vi "SubMain1_WriteEEPROM_vna_wmg.vi"(6 "Date":u8[](array[numeric])=[49, 53, 48, 56, 50, 52] format="%.0x", 7 "VendorSN":u8[](array[numeric])=[49, 53, 50, 51, 54, 48, 48, 48, 53] format="%.0x", 8 "PN":string="H3C QSFP+", 9 "命令类型选择":string="H3C QSFP+", 10 "local":bool, 11 "VISA resource name":refnum<visa-resource-name>="COM1") -> (0 "cmd_input":string[][](array[string]), 1 "readout":string[][](array[string]), 2 "readout":u8[][](array[numeric]) format="%.0x", 3 "info_write":string[][](array[string]), 4 "type_array":string[](array[string]), 5 "exist?":bool)   [LabVIEW 2011]
uses:
  <vilib>/Utility/file.llb/Read From Spreadsheet File (string).vi
panel:
  out "output":string[][](array[string])
  out "电子表格字符串":string
  out "ext_array":string[][](array[string])
  out "ref_random":refnum<vi>
  in  "random":string[](array[string])
  out "ref_channel":refnum<vi>
  in  "channel":i8
  out "EEPROM_OK?":bool[](array[boolean])
  out "message":string
  # "EEPROM Information Output"
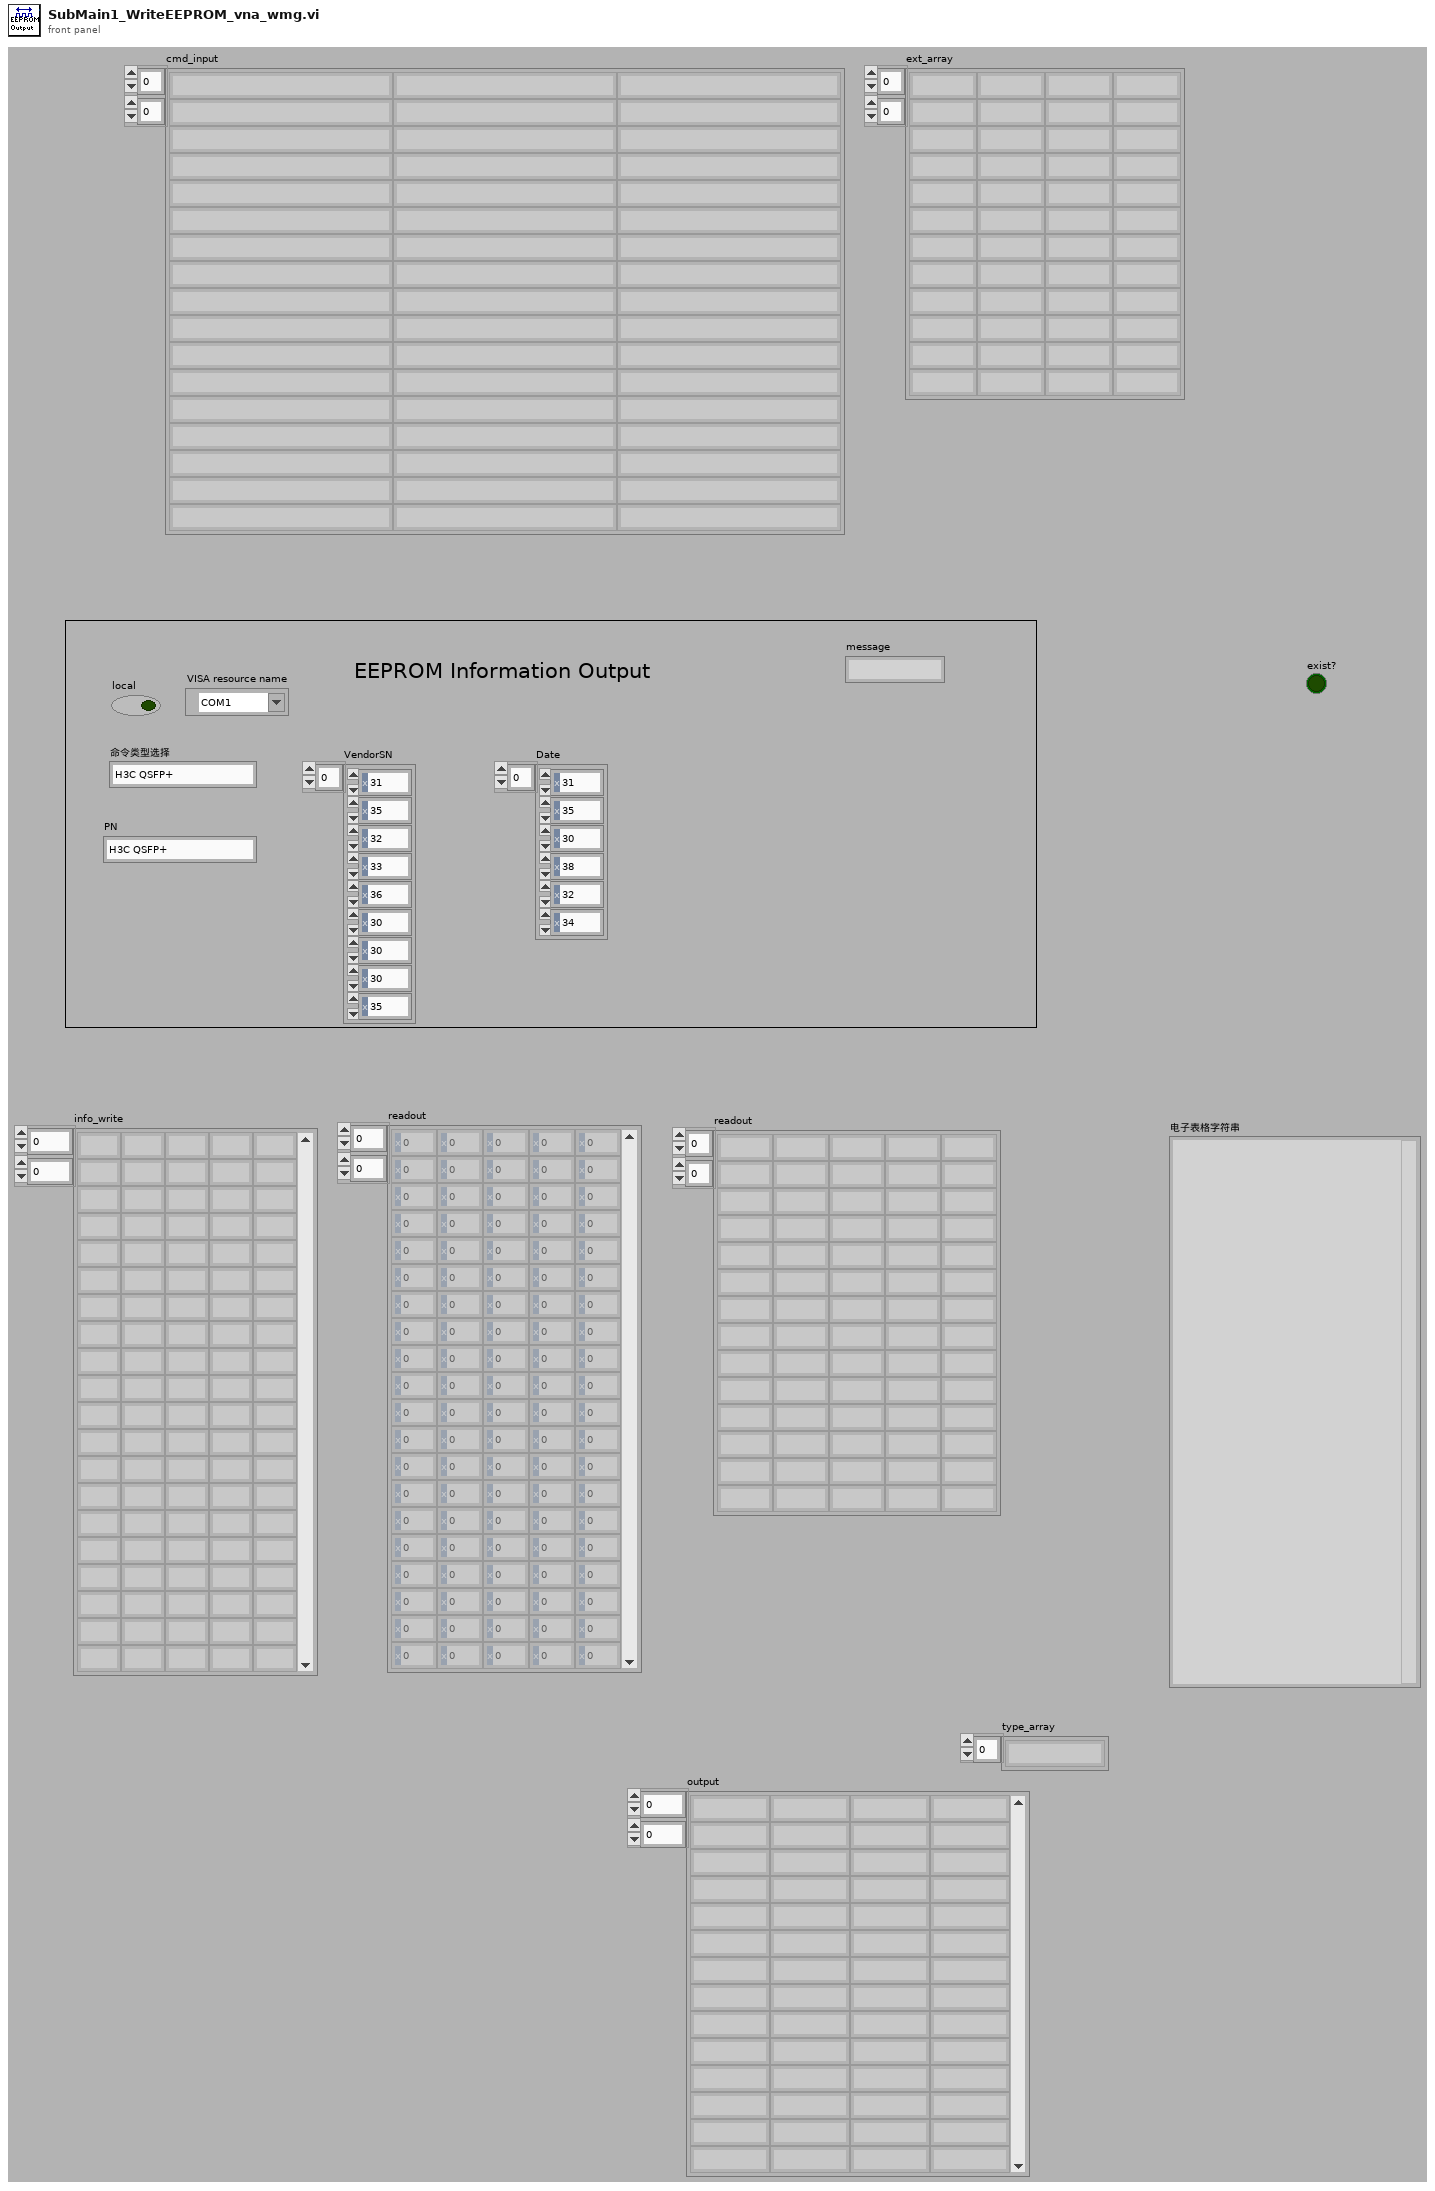
[diagram p1: front panel]
types:
  T1 = enum16{"查询表名", "查询列名", "查询记录", "查询总记录", "查询数据", "转换数据"}
  T2 = enum16{"big-endian, network order", "native, host order", "little-endian"}
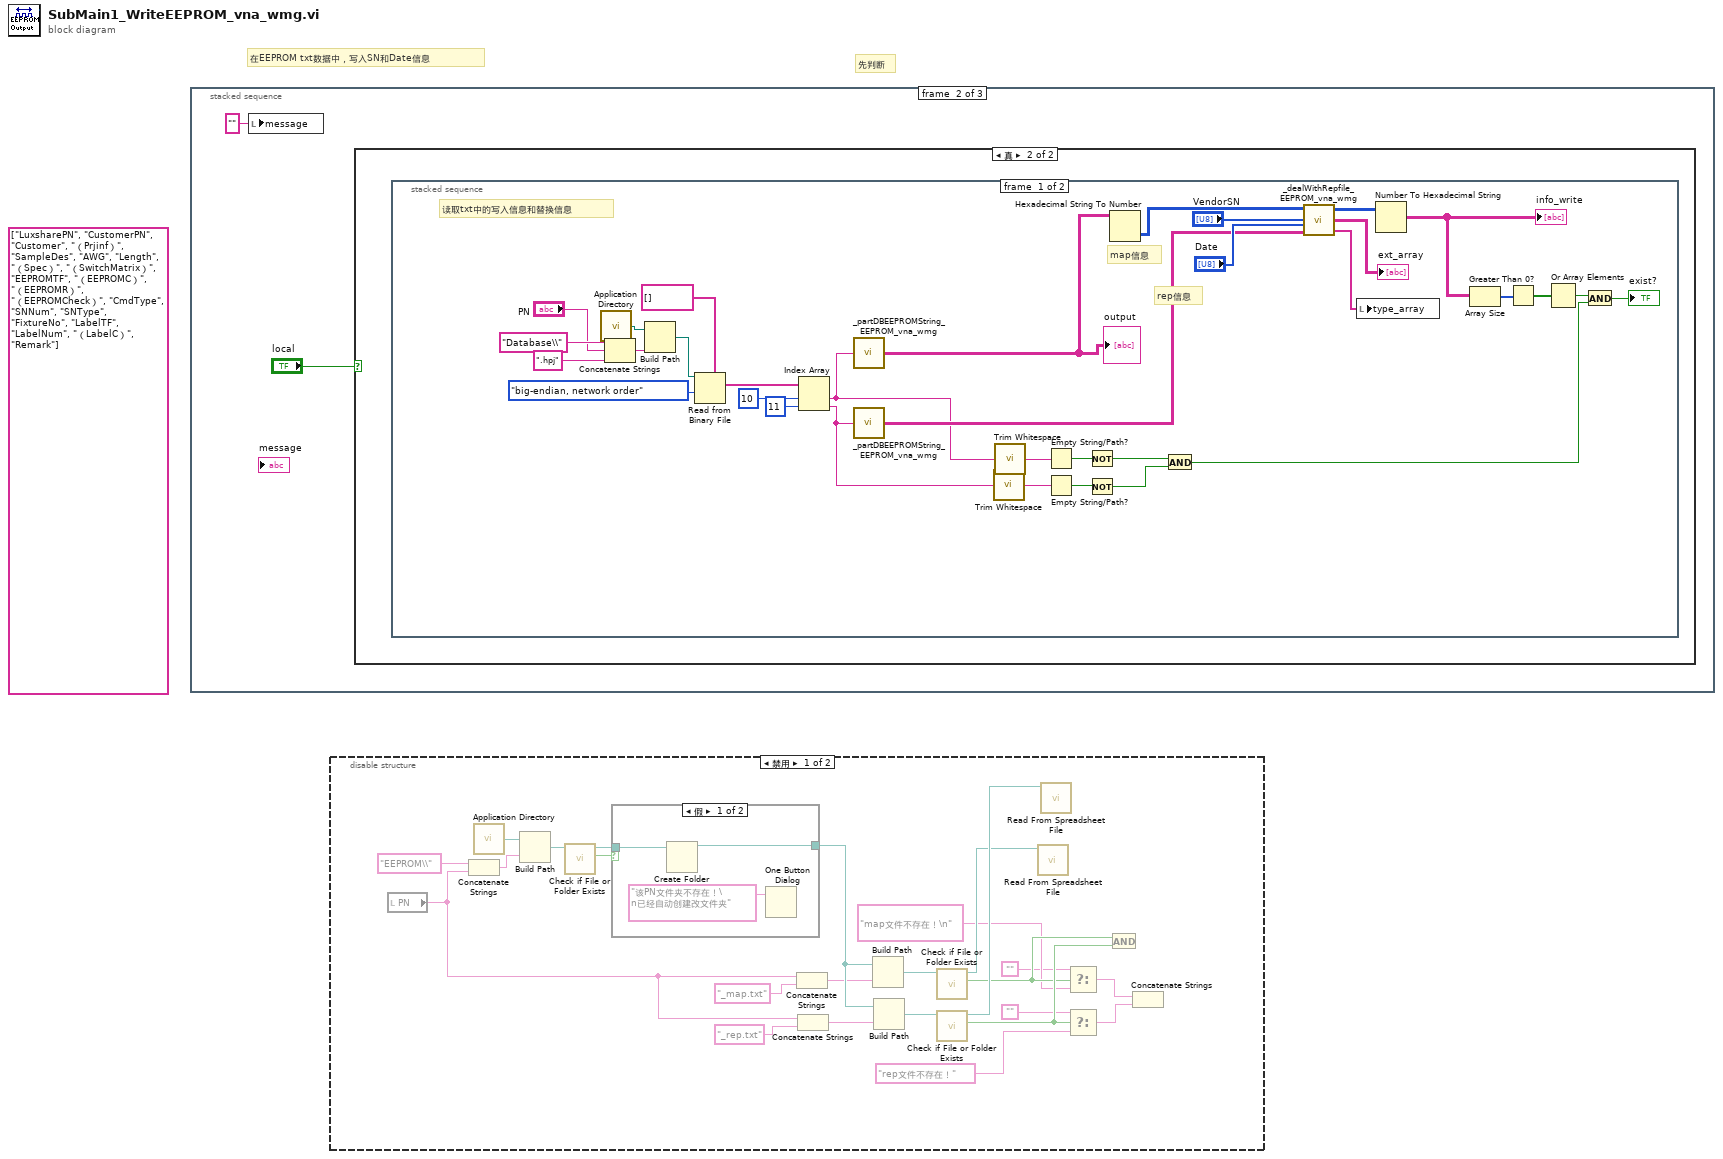
[diagram p0: block diagram]
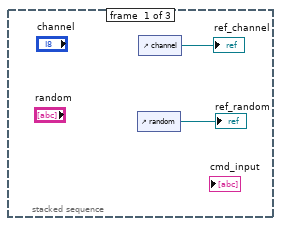
[diagram p4: hidden frame]
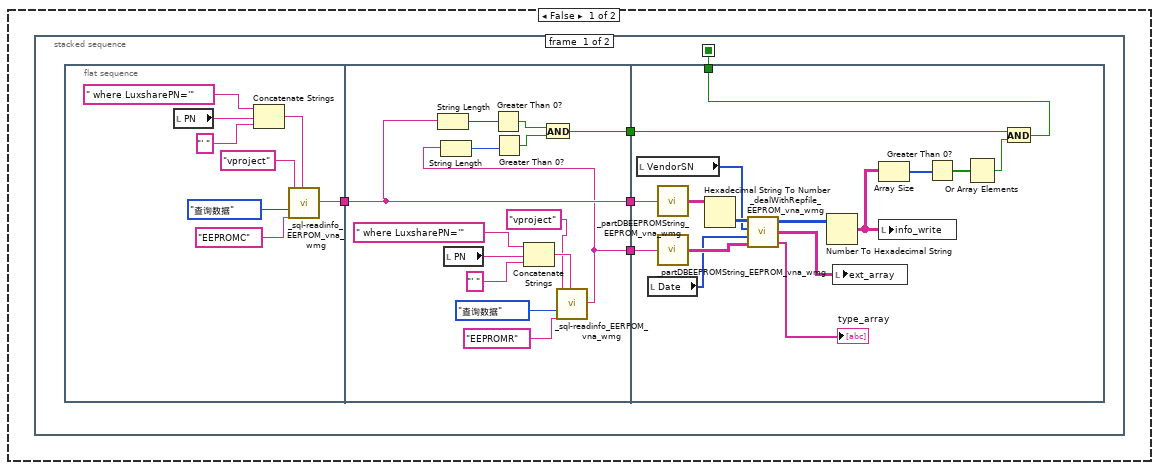
[diagram p5: hidden frame]
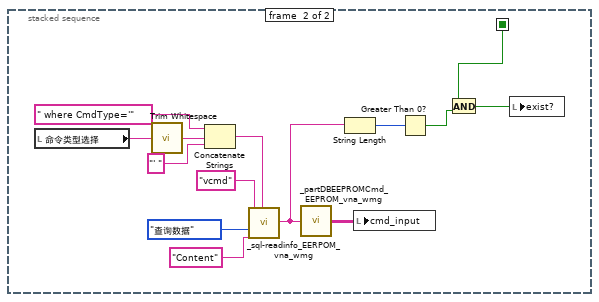
[diagram p6: hidden frame]
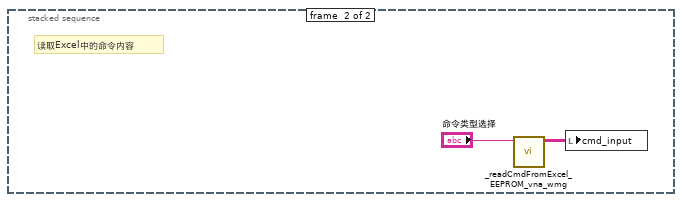
[diagram p7: hidden frame]
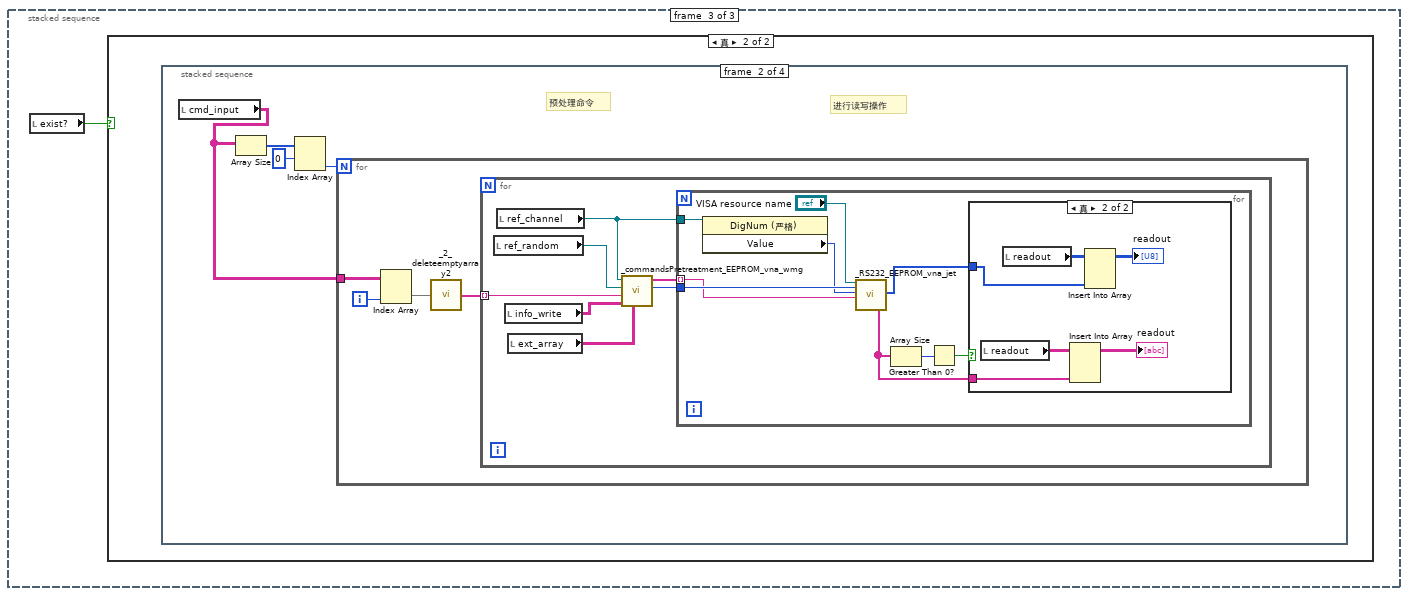
[diagram p8: hidden frame]
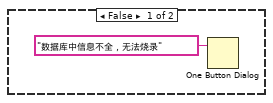
[diagram p9: hidden frame]
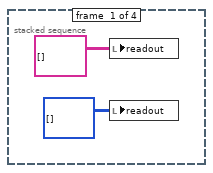
[diagram p10: hidden frame]
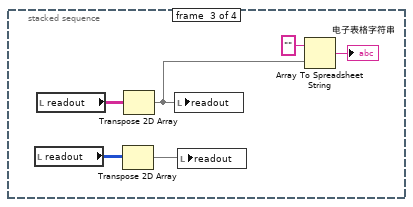
[diagram p12: hidden frame]
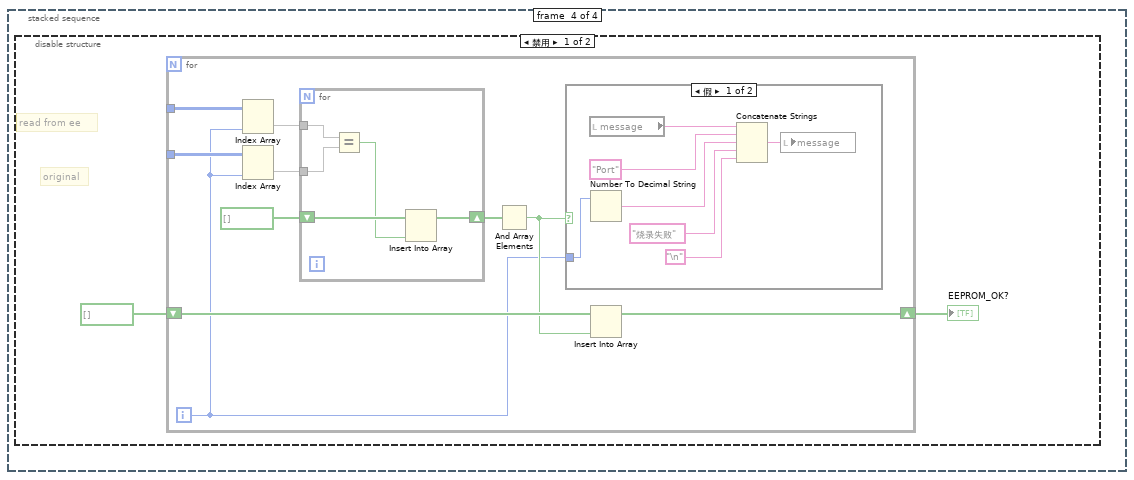
[diagram p13: hidden frame]
diagram:
  (unwired) string[] ["LuxsharePN", "CustomerPN", "Customer", "（Prjinf）", "SampleDes", "AWG", "Length", "（Spec）", "（SwitchMatrix）", "EEPROMTF", "（EEPROMC）", "（EEPROMR）", "（EEPROMCheck）", "CmdType", "SNNum", "SNType", "FixtureNo", "LabelTF", "LabelNum", "（LabelC）", "Remark"] ("列名")
  # "在EEPROM txt数据中，写入SN和Date信息"
  # "先判断"
  n1 = stacked-sequence {
    frame #0 {
      n2 = control-ref of="random"() -> (→"ref_random":refnum<vi>)
      n3 = control-ref of="channel"() -> (→"ref_channel":refnum<vi>)
    }
    frame #1 {
      n4 = local write "message"("" ("message")) -> ()
      n5 = case shown="真" "local" {
        frame False {
          n6 = stacked-sequence {
            seq-local: [w5 _] -> [_ w49]
            frame #0 {
              n7 = flat-sequence {
                tunnel: [w11] -> w9
                tunnel: w9 -> [w25]
                tunnel: [w25] -> w8
                tunnel: [w24] -> w7
                tunnel: [w19] -> w6
                tunnel: w8 -> [w47]
                tunnel: w7 -> [w46]
                tunnel: w6 -> [w37]
                tunnel: [w36] -> w5
                frame #0 {
                  n8 = local read "PN"() -> (w16:string)
                  n9 = Concatenate Strings(" where LuxsharePN='", w16, "' ") -> (w13:string)
                  n10 = call "_sql-readinfo_EERPOM_vna_wmg.vi"("操作模式"=T1."查询数据", "查询项目"="EEPROMC", "表名"="vproject", "限定条件"=w13) -> ("ResultString"=w11:string)  [unwired: 13 in, 10 out]
                }
                frame #1 {
                  n11 = String Length(string=w25) -> (length=w23:i32)
                  n12 = local read "PN"() -> (w27:string)
                  n13 = Greater Than 0?(x=w23) -> (x > 0?=w21:bool)
                  n14 = Concatenate Strings(" where LuxsharePN='", w27, "' ") -> (w30:string)
                  n15 = call "_sql-readinfo_EERPOM_vna_wmg.vi"("操作模式"=T1."查询数据", "查询项目"="EEPROMR", "表名"="vproject", "限定条件"=w30) -> ("ResultString"=w24:string)  [unwired: 13 in, 10 out]
                  n16 = String Length(string=w24) -> (length=w22:i32)
                  n17 = Greater Than 0?(x=w22) -> (x > 0?=w20:bool)
                  n18 = And(x=w21, y=w20) -> (x .and. y?=w19:bool)
                }
                frame #2 {
                  n19 = local read "VendorSN"() -> (w40:u8[])
                  n20 = local read "Date"() -> (w39:u8[])
                  n21 = call "_partDBEEPROMString_EEPROM_vna_wmg.vi"("input"=w47) -> ("output"=w44:string[][])
                  n22 = call "_partDBEEPROMString_EEPROM_vna_wmg.vi"("input"=w46) -> ("output"=w42:string[][])
                  n23 = Hexadecimal String To Number(string=w44) -> (number=w43:u32[][])  [unwired: 2 in, 1 out]
                  n24 = call "_dealWithRepfile_EEPROM_vna_wmg.vi"("eeprom_map"=w43, "VendorSN"=w40, "Date"=w39, "eeprom_rep"=w42) -> ("eeprom_map_out"=w45:u8[][], "ext_array"=w41:string[][], "type_array"=→"type_array":string[])  [unwired: 1 in]
                  n25 = Number To Hexadecimal String(2:w45) -> (0:w35:string[][])  [unwired: 1 in]
                  n26 = local write "ext_array"(w41) -> ()
                  n27 = Array Size(array=w35) -> (size(s)=w34:i32[])
                  n28 = local write "info_write"(w35) -> ()
                  n29 = Greater Than 0?(x=w34) -> (x > 0?=w33:bool[])
                  n30 = Or Array Elements(Boolean array=w33) -> (logical OR=w32:bool)
                  n31 = And(x=w37, y=w32) -> (x .and. y?=w36:bool)
                }
              }
            }
            frame #1 {
              n32 = local read "命令类型选择"() -> (w54:string)
              n33 = call <vilib>:"Trim Whitespace.vi"("string"=w54) -> ("trimmed string"=w55:string)  [unwired: 1 in]
              n34 = Concatenate Strings(" where CmdType='", w55, "' ") -> (w60:string)
              n35 = call "_sql-readinfo_EERPOM_vna_wmg.vi"("操作模式"=T1."查询数据", "查询项目"="Content", "表名"="vcmd", "限定条件"=w60) -> ("ResultString"=w52:string)  [unwired: 13 in, 10 out]
              n36 = call "_partDBEEPROMCmd_EEPROM_vna_wmg.vi"("input"=w52) -> ("output"=w53:string[][])
              n37 = String Length(string=w52) -> (length=w51:i32)
              n38 = local write "cmd_input"(w53) -> ()
              n39 = Greater Than 0?(x=w51) -> (x > 0?=w50:bool)
              n40 = And(x=w49, y=w50) -> (x .and. y?=w48:bool)
              n41 = local write "exist?"(w48) -> ()
            }
          }
        }
        frame True {
          n42 = stacked-sequence {
            frame #0 {
              # "map信息"
              # "rep信息"
              # "读取txt中的写入信息和替换信息"
              n43 = call <vilib>:"Application Directory.vi"() -> ("Application Directory"=w76:path)
              n44 = Concatenate Strings("Database\\" ("字符串"), "PN", ".hpj" ("字符串")) -> (w77:string)
              n45 = Build Path(base path=w76, name or relative path=w77) -> (appended path=w82:path)
              n46 = Read from Binary File(5:string[] [], 9:T2."big-endian, network order" ("字节顺序(0:big-endian, network order)"), 11:w82) -> (2:w83:string[])  [unwired: 3 in, 3 out]
              n47 = Index Array(array=w83, index #1=10 ("索引"), index #2=11 ("索引")) -> (element #1=w69:string, element #2=w68:string)
              n48 = call "_partDBEEPROMString_EEPROM_vna_wmg.vi"("input"=w69) -> ("output"=w62:string[][])
              "output" <- w62
              n49 = call "_partDBEEPROMString_EEPROM_vna_wmg.vi"("input"=w68) -> ("output"=w72:string[][])
              n50 = call <vilib>:"Trim Whitespace.vi"("string"=w68) -> ("trimmed string"=w70:string)  [unwired: 1 in]
              n51 = call <vilib>:"Trim Whitespace.vi"("string"=w69) -> ("trimmed string"=w71:string)  [unwired: 1 in]
              n52 = Empty String/Path?(string/path=w71) -> (empty?=w67:bool)
              n53 = Empty String/Path?(string/path=w70) -> (empty?=w66:bool)
              n54 = Not(x=w67) -> (.not. x?=w65:bool)
              n55 = Not(x=w66) -> (.not. x?=w64:bool)
              n56 = Hexadecimal String To Number(string=w62) -> (number=w84:u32[][])  [unwired: 2 in, 1 out]
              n57 = And(x=w65, y=w64) -> (x .and. y?=w63:bool)
              n58 = call "_dealWithRepfile_EEPROM_vna_wmg.vi"("eeprom_map"=w84, "VendorSN"="VendorSN", "Date"="Date", "eeprom_rep"=w72) -> ("eeprom_map_out"=w94:u8[][], "ext_array"=→"ext_array":string[][], "type_array"=w90:string[])  [unwired: 1 in]
              n59 = local write "type_array"(w90) -> ()
              n60 = Number To Hexadecimal String(2:w94) -> (0:w85:string[][])  [unwired: 1 in]
              "info_write" <- w85
              n61 = Array Size(array=w85) -> (size(s)=w88:i32[])
              n62 = Greater Than 0?(x=w88) -> (x > 0?=w87:bool[])
              n63 = Or Array Elements(Boolean array=w87) -> (logical OR=w86:bool)
              n64 = And(x=w86, y=w63) -> (x .and. y?=→"exist?":bool)
            }
            frame #1 {
              # "读取Excel中的命令内容"
              n65 = call "_readCmdFromExcel_EEPROM_vna_wmg.vi"("命令类型选择"="命令类型选择") -> ("cmd"=w95:string[][])  [unwired: 10 in]
              n66 = local write "cmd_input"(w95) -> ()
            }
          }
        }
      }
    }
    frame #2 {
      n67 = local read "exist?"() -> (w97:bool)
      n68 = case shown="真" w97 {
        frame False {
          n69 = One Button Dialog(message="数据库中信息不全，无法烧录" ("消息")) -> ()  [unwired: 1 in, 1 out]
        }
        frame True {
          n70 = stacked-sequence {
            frame #0 {
              n71 = local write "readout"(string[][] []) -> ()
              n72 = local write "readout"(u8[][] [] ("readout")) -> ()
            }
            frame #1 {
              # "进行读写操作"
              # "预处理命令"
              n73 = local read "cmd_input"() -> (w101:string[][])
              n74 = Array Size(array=w101) -> (size(s)=w104:i32[])
              n75 = Index Array(array=w104, index #1=0 ("索引")) -> (element #2=w102:i32)  [unwired: 1 in, 1 out]
              n76 = for {
                N: w102 -> [_]
                tunnel: w101 -> [w108]
                i -> [w107]
                n77 = Index Array(array=w108, index (col)=w107) -> (element=w106:string[])  [unwired: 1 in]
                n78 = call "_2_deleteemptyarray2.vi"("input"=w106) -> ("in_cons"=w105:string[])
                n79 = for {
                  tunnel: w105 -> [w113] mode=indexing
                  n80 = local read "ref_random"() -> (w114:refnum<vi>)
                  n81 = local read "ref_channel"() -> (w111:refnum<vi>)
                  n82 = local read "info_write"() -> (w110:string[][])
                  n83 = local read "ext_array"() -> (w109:string[][])
                  n84 = call "_commandsPretreatment_EEPROM_vna_wmg.vi"("array1_input"=w109, "array0_input"=w110, "cmd_input"=w113, "ref_random"=w114, "ref_channel"=w111) -> ("Function"=w112:enum16{"Write to EEPROM", "Read From EEPROM"}, "cmd_output"=w115:string[])  [unwired: 5 in]
                  n85 = for {
                    tunnel: w115 -> [w123] mode=indexing
                    tunnel: w112 -> [w124]
                    tunnel: w111 -> [w122]
                    n86 = property class="DigNum (严格)"(reference=w122) -> ("Value"=w121:i8)  [unwired: 1 in, 2 out]
                    n87 = call "_RS232_EEPROM_vna_jet.vi"("VISA resource name"="VISA resource name", "Function"=w124, "Select channel"=w121, "input_cmd"=w123) -> (13:"readout"=w117:string[], 16:"readout"=w116:u8[])  [unwired: 9 in, 5 out]
                    n88 = Array Size(array=w117) -> (size(s)=w119:i32)
                    n89 = Greater Than 0?(x=w119) -> (x > 0?=w118:bool)
                    n90 = case shown="真" w118 {
                      tunnel: w117 -> [_ w129]
                      tunnel: w116 -> [_ w126]
                      frame False {
                      }
                      frame True {
                        n91 = local read "readout"() -> (w130:string[][])
                        n92 = local read "readout"() -> (w127:u8[][])
                        n93 = Insert Into Array(array=w130, new element=w129) -> (→"readout":string[][])  [unwired: 2 in]
                        n94 = Insert Into Array(array=w127, new element=w126) -> (→"readout":u8[][])  [unwired: 2 in]
                      }
                    }
                  }
                }
              }
            }
            frame #2 {
              n95 = local read "readout"() -> (w135:u8[][])
              n96 = local read "readout"() -> (w136:string[][])
              n97 = Transpose 2D Array(2D array=w135) -> (transposed array=w134:u8[][])
              n98 = Transpose 2D Array(2D array=w136) -> (transposed array=w133:string[][])
              n99 = local write "readout"(w133) -> ()
              n100 = local write "readout"(w134) -> ()
              n101 = Array To Spreadsheet String(array=w133, 3:"" ("格式字符串")) -> (spreadsheet string=→"电子表格字符串":string)  [unwired: 1 in]
            }
            frame #3 {
              n102 = disable-structure shown="禁用" {
                frame Disabled {
                  # "read from ee"
                  # "original"
                  n103 = for {
                    N: [_] -> w141
                    tunnel: [w151] -> w140
                    tunnel: [w150] -> w139
                    shift-right: [w144] -> w137
                    shift-left: bool[] [] -> [w145]
                    i -> [w142]
                    n104 = Index Array(array=w151, index (col)=w142) -> (element=w149)  [unwired: 1 in]
                    n105 = Index Array(array=w150, index (col)=w142) -> (element=w148)  [unwired: 1 in]
                    n106 = for {
                      tunnel: w149 -> [w163]
                      tunnel: w148 -> [w162]
                      shift-right: [w159] -> w146
                      shift-left: bool[] [] -> [w161]
                      n107 = Equal?(x=w163, y=w162) -> (x = y?=w160:bool)
                      n108 = Insert Into Array(array=w161, new element=w160) -> (w159:bool[])  [unwired: 1 in]
                    }
                    n109 = And Array Elements(Boolean array=w146) -> (logical AND=w143:bool)
                    n110 = case shown="假" w143 {
                      tunnel: w142 -> [w157 _]
                      frame False {
                        n111 = local read "message"() -> (w158:string)
                        n112 = Number To Decimal String(number=w157) -> (decimal integer string=w155:string)  [unwired: 1 in]
                        n113 = Concatenate Strings(w158, "Port", w155, "烧录失败", "\n") -> (w152:string)
                        n114 = local write "message"(w152) -> ()
                      }
                      frame True {
                      }
                    }
                    n115 = Insert Into Array(array=w145, new element=w143) -> (w144:bool[])  [unwired: 1 in]
                  }
                  "EEPROM_OK?" <- w137
                }
                frame Enabled {
                }
              }
            }
          }
        }
      }
    }
  }
  n116 = disable-structure shown="禁用" {
    frame Disabled {
      n117 = local read "PN"() -> (w187:string)
      n118 = Concatenate Strings("EEPROM\\", w187) -> (w165:string)
      n119 = call <vilib>:"Application Directory.vi"() -> ("Application Directory"=w173:path)
      n120 = Build Path(base path=w173, name or relative path=w165) -> (appended path=w166:path)
      n121 = call <vilib>:"Check if File or Folder Exists.vi"("path"=w166) -> ("file or folder exists?"=w167:bool, "dup path"=w168:path)  [unwired: 8 in, 1 out]
      n122 = case shown="假" w167 {
        tunnel: w168 -> [w189 w191]
        tunnel: [w188 w191] -> w176
        frame False {
          n123 = Create Folder(path (use dialog)=w189) -> (created path=w188:path)  [unwired: 2 in, 2 out]
          n124 = One Button Dialog(message="该PN文件夹不存在！\n已经自动创建改文件夹" ("消息")) -> ()  [unwired: 1 in, 1 out]
        }
        frame True {
        }
      }
      n125 = Concatenate Strings(w187, "_map.txt" ("字符串")) -> (w171:string)
      n126 = Concatenate Strings(w187, "_rep.txt" ("字符串")) -> (w172:string)
      n127 = Build Path(base path=w176, name or relative path=w171) -> (appended path=w174:path)
      n128 = Build Path(base path=w176, name or relative path=w172) -> (appended path=w175:path)
      n129 = call <vilib>:"Check if File or Folder Exists.vi"("path"=w174) -> ("file or folder exists?"=w183:bool, "dup path"=w185:path)  [unwired: 8 in, 1 out]
      n130 = call <vilib>:"Check if File or Folder Exists.vi"("path"=w175) -> ("file or folder exists?"=w184:bool, "dup path"=w186:path)  [unwired: 8 in, 1 out]
      n131 = call-poly <vilib>:"Read From Spreadsheet File.vi"("file path (dialog if empty)"=w185) -> ()  [unwired: 6 in, 5 out]
      n132 = call-poly <vilib>:"Read From Spreadsheet File.vi"("file path (dialog if empty)"=w186) -> ()  [unwired: 6 in, 5 out]
      n133 = Select(t="", s=w183, f="map文件不存在！\n") -> (s? t:f=w181:string)
      n134 = Select(t="", s=w184, f="rep文件不存在！") -> (s? t:f=w182:string)
      n135 = And(x=w183, y=w184) -> ()  [unwired: 1 out]
      n136 = Concatenate Strings(w181, w182) -> ()  [unwired: 1 out]
    }
    frame Enabled {
    }
  }
